vi "Polynomial Plot.vi"   [LabVIEW 2020, in "NI_AALPro.lvlib"]
doc: "Plots the evaluations of polynomial <B>P(x)</B>. Wire data to the <B>X</B> input to determine the polymorphic instance to use or manually select the instance."
uses:
  NI_AALPro.lvlib
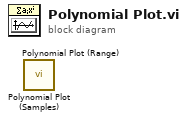
[diagram p0: block diagram]
diagram:
  n1 = call "Polynomial Plot (Samples).vi"() -> ()  [unwired: 10 in, 2 out]
  n2 = call "Polynomial Plot (Range).vi"() -> ()  [unwired: 10 in, 2 out]
